vi "SawRawStatistics.vi"(7 "elements 2":cluster{"Intensity Graph 3":u8[][]}[](array[cluster]), 8 "error in (no error)":errorcluster, 11 "Full File Path":path) -> (0 "error out":errorcluster)   [LabVIEW 2018, in "statistics.lvlib"]
uses:
  statistics.lvlib
  Read and Save Files/RW_Protocols.lvlib
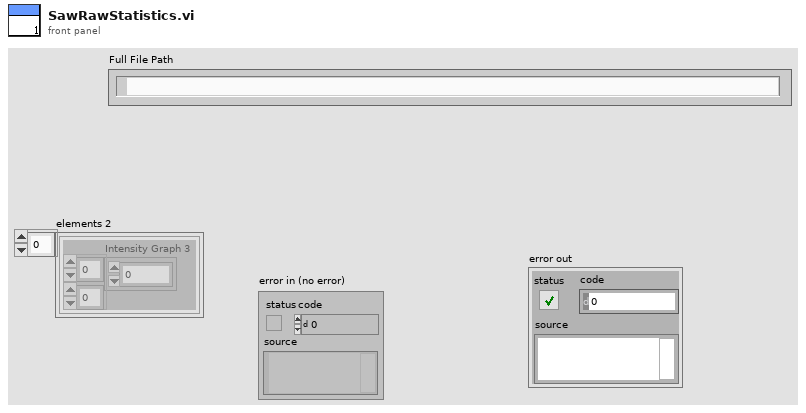
[diagram p1: front panel]
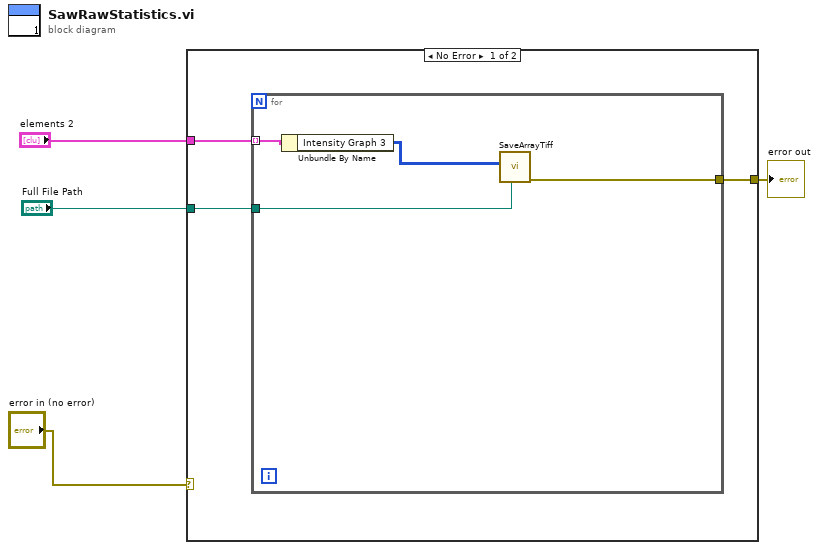
[diagram p0: block diagram]
diagram:
  n1 = case shown="No Error" "error in (no error)" {
    selector: "error in (no error)" -> [_ w12]
    tunnel: "elements 2" -> [w7 _]
    tunnel: "Full File Path" -> [w6 _]
    tunnel: [w5 w12] -> w1
    frame No Error {
      n2 = for {
        tunnel: w7 -> [w11] mode=indexing
        tunnel: w6 -> [w9]
        tunnel: [w8] -> w5
        n3 = Unbundle By Name(w11) -> ("Intensity Graph 3"=w10:u8[][])
        n4 = call "SaveArrayTiff.vi"("Target Folder"=w9, "output array"=w10) -> ("error out"=w8:errorcluster)  [unwired: 9 in]
      }
    }
    frame Error {
    }
  }
  "error out" <- w1
